vi "一致性结果判定.vi"() -> (14 "1":bool=TRUE, 15 "2":bool=TRUE, 16 "3":bool=TRUE, 17 "4":bool=TRUE, 18 "5":bool=TRUE, 19 "6":bool=TRUE)   [LabVIEW 2017]
panel:
  out "添加的数组 2":u32[](array[numeric])
  out "数组":bool[](array[boolean])
  in  "位置范围设定":T1={"位置1"={"上限"=726.0, "下限"=686.0}, "位置2"={"上限"=874.0, "下限"=834.0}, "位置3"={"上限"=997.0, "下限"=957.0}, "位置4"={"上限"=1139.0, "下限"=1099.0}, "位置5"={"上限"=1283.0, "下限"=1243.0}, "位置6"={"上限"=1429.0, "下限"=1389.0}, "位置7"={"上限"=1576.0, "下限"=1536.0}, "位置8"={"上限"=1728.0, "下限"=1688.0}, "位置9"={"上限"=1879.0, "下限"=1839.0}, "位置10"={"上限"=2036.0, "下限"=1996.0}}
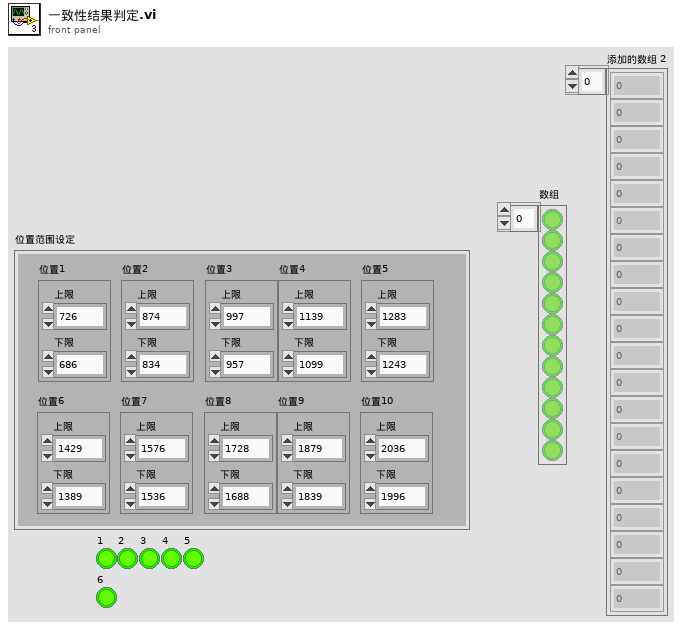
[diagram p1: front panel]
types:
  T1 = cluster{"位置1":cluster{"上限":dbl, "下限":dbl}, "位置2":cluster{"上限":dbl, "下限":dbl}, "位置3":cluster{"上限":dbl, "下限":dbl}, "位置4":cluster{"上限":dbl, "下限":dbl}, "位置5":cluster{"上限":dbl, "下限":dbl}, "位置6":cluster{"上限":dbl, "下限":dbl}, "位置7":cluster{"上限":dbl, "下限":dbl}, "位置8":cluster{"上限":dbl, "下限":dbl}, "位置9":cluster{"上限":dbl, "下限":dbl}, "位置10":cluster{"上限":dbl, "下限":dbl}}
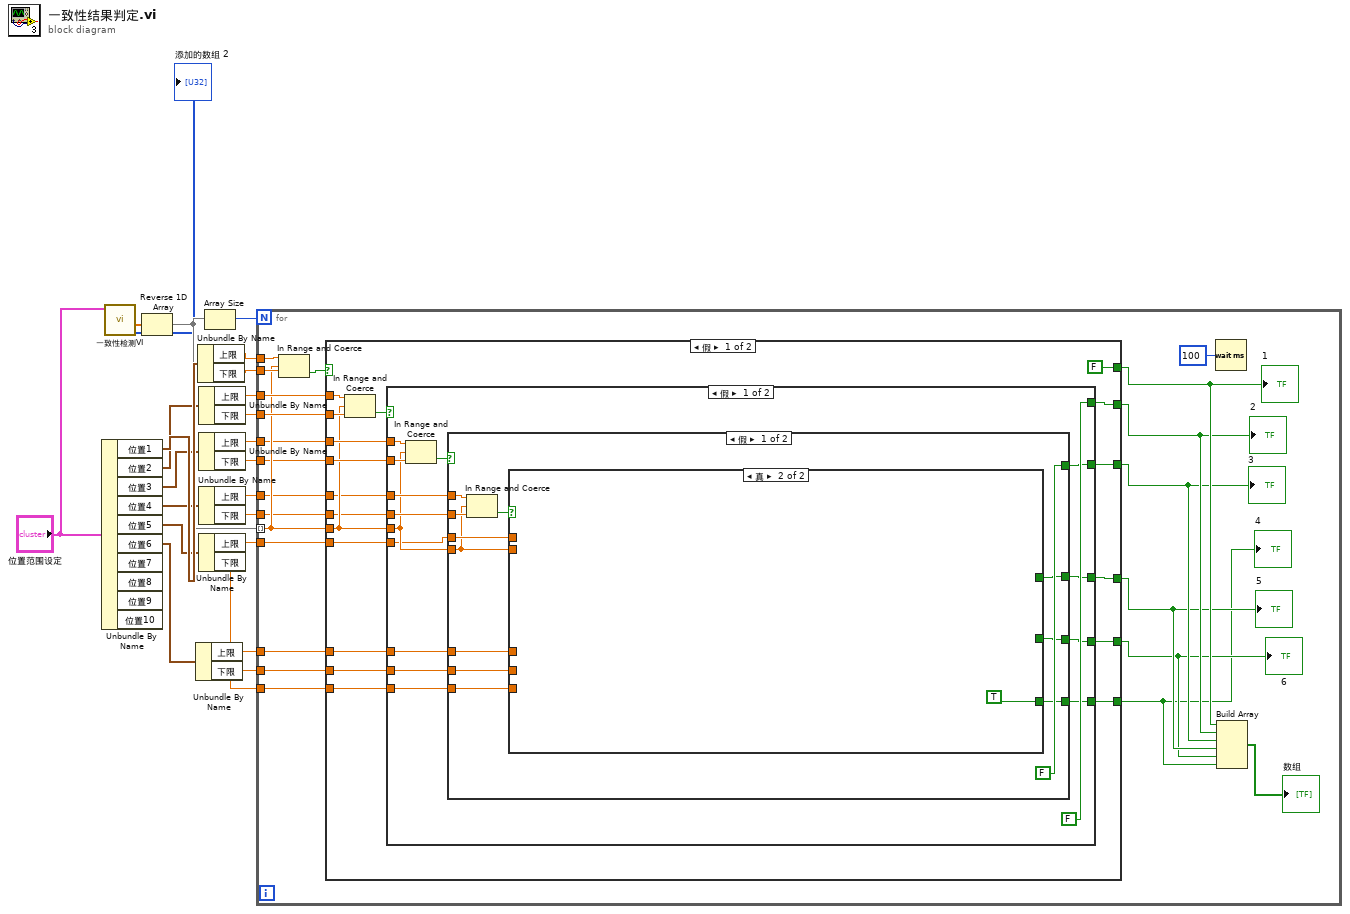
[diagram p0: block diagram]
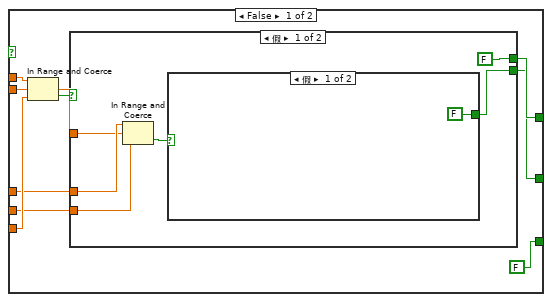
[diagram p2: hidden frame]
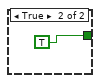
[diagram p3: hidden frame]
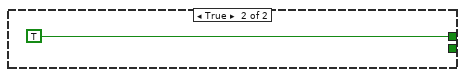
[diagram p4: hidden frame]
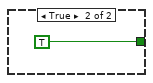
[diagram p5: hidden frame]
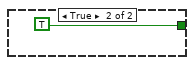
[diagram p6: hidden frame]
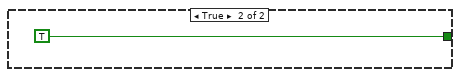
[diagram p7: hidden frame]
diagram:
  n1 = Unbundle By Name("位置范围设定") -> ("位置1"=w23:cluster{"上限":dbl, "下限":dbl}, "位置2"=w18:cluster{"上限":dbl, "下限":dbl}, "位置3"=w15:cluster{"上限":dbl, "下限":dbl}, "位置4"=w12:cluster{"上限":dbl, "下限":dbl}, "位置5"=w9:cluster{"上限":dbl, "下限":dbl}, "位置6"=w6:cluster{"上限":dbl, "下限":dbl})  [unwired: 4 out]
  n2 = call "一致性检测VI.vi"("位置范围设定"="位置范围设定") -> ("添加的数组 2"=→"添加的数组 2":u32[], "添加的数组"=w21:sgl[])  [unwired: 7 in, 2 out]
  n3 = Reverse 1D Array(array=w21) -> (reversed array=w2:sgl[])
  n4 = Unbundle By Name(w6) -> ("上限"=w5:dbl, "下限"=w4:dbl)
  n5 = Unbundle By Name(w23) -> ("上限"=w19:dbl, "下限"=w20:dbl)
  n6 = Unbundle By Name(w18) -> ("上限"=w16:dbl, "下限"=w17:dbl)
  n7 = Unbundle By Name(w15) -> ("上限"=w14:dbl, "下限"=w13:dbl)
  n8 = Unbundle By Name(w12) -> ("上限"=w11:dbl, "下限"=w10:dbl)
  n9 = Unbundle By Name(w9) -> ("上限"=w8:dbl, "下限"=w7:dbl)
  n10 = Array Size(array=w2) -> (size(s)=w22:i32)
  n11 = for {
    N: w22 -> [_]
    tunnel: w2 -> [w40] mode=indexing
    tunnel: w20 -> [w45]
    tunnel: w19 -> [w44]
    tunnel: w17 -> [w42]
    tunnel: w16 -> [w41]
    tunnel: w14 -> [w39]
    tunnel: w13 -> [w38]
    tunnel: w11 -> [w37]
    tunnel: w10 -> [w36]
    tunnel: w8 -> [w35]
    tunnel: w7 -> [w34]
    tunnel: w5 -> [w33]
    tunnel: w4 -> [w32]
    n12 = In Range and Coerce(upper limit=w44, x=w40, lower limit=w45) -> (In Range?=w43:bool)  [unwired: 1 out]
    n13 = case shown="假" w43 {
      tunnel: [FALSE ("1") TRUE ("1")] -> w30
      tunnel: w42 -> [w62 _]
      tunnel: w41 -> [w61 _]
      tunnel: w40 -> [w56 _]
      tunnel: [w59 _] -> w29
      tunnel: w39 -> [w58 _]
      tunnel: w38 -> [w57 _]
      tunnel: [w55 _] -> w28
      tunnel: w37 -> [w54 _]
      tunnel: w36 -> [w53 _]
      tunnel: [w52 _] -> w25
      tunnel: w35 -> [w51 _]
      tunnel: w34 -> [w50 _]
      tunnel: [w49 _] -> w27
      tunnel: w33 -> [w48 _]
      tunnel: w32 -> [w47 _]
      tunnel: [w46 _] -> w26
      frame False {
        n14 = In Range and Coerce(upper limit=w61, x=w56, lower limit=w62) -> (In Range?=w60:bool)  [unwired: 1 out]
        n15 = case shown="假" w60 {
          tunnel: [FALSE TRUE] -> w59
          tunnel: w58 -> [w76 _]
          tunnel: w57 -> [w75 _]
          tunnel: w56 -> [w71 _]
          tunnel: [w74 _] -> w55
          tunnel: w54 -> [w73 _]
          tunnel: w53 -> [w72 _]
          tunnel: [w70 _] -> w52
          tunnel: w51 -> [w69 _]
          tunnel: w50 -> [w68 _]
          tunnel: [w67 _] -> w49
          tunnel: w48 -> [w66 _]
          tunnel: w47 -> [w65 _]
          tunnel: [w64 _] -> w46
          frame False {
            n16 = In Range and Coerce(upper limit=w76, x=w71, lower limit=w75) -> (In Range?=w77:bool)  [unwired: 1 out]
            n17 = case shown="假" w77 {
              tunnel: [FALSE TRUE] -> w74
              tunnel: w73 -> [w88 _]
              tunnel: w72 -> [w87 _]
              tunnel: w71 -> [w82 _]
              tunnel: [w86 _] -> w70
              tunnel: w69 -> [w85 _]
              tunnel: w68 -> [w84 _]
              tunnel: [w83 _] -> w67
              tunnel: w66 -> [w81 _]
              tunnel: w65 -> [w80 _]
              tunnel: [w79 _] -> w64
              frame False {
                n18 = In Range and Coerce(upper limit=w88, x=w82, lower limit=w87) -> (In Range?=w89:bool)  [unwired: 1 out]
                n19 = case shown="真" w89 {
                  tunnel: [FALSE TRUE] -> w86
                  tunnel: w85 -> [w97 _]
                  tunnel: w84 -> [w96 _]
                  tunnel: [w95 _] -> w83
                  tunnel: w82 -> [w92 _]
                  tunnel: w81 -> [w94 _]
                  tunnel: w80 -> [w93 _]
                  tunnel: [w91 _] -> w79
                  frame False {
                    n20 = In Range and Coerce(upper limit=w97, x=w92, lower limit=w96) -> (In Range?=w98:bool)  [unwired: 1 out]
                    n21 = case shown="假" w98 {
                      tunnel: [FALSE TRUE] -> w95
                      tunnel: w94 -> [w103 _]
                      tunnel: w93 -> [w102 _]
                      tunnel: w92 -> [w101 _]
                      tunnel: [w100 _] -> w91
                      frame False {
                        n22 = In Range and Coerce(upper limit=w103, x=w101, lower limit=w102) -> (In Range?=w104:bool)  [unwired: 1 out]
                        n23 = case shown="假" w104 {
                          tunnel: [FALSE TRUE] -> w100
                          frame False {
                          }
                          frame True {
                          }
                        }
                      }
                      frame True {
                      }
                    }
                  }
                  frame True {
                  }
                }
              }
              frame True {
              }
            }
          }
          frame True {
          }
        }
      }
      frame True {
      }
    }
    "1" <- w30
    "2" <- w29
    "3" <- w28
    "4" <- w25
    "5" <- w27
    "6" <- w26
    n24 = Wait (ms)(milliseconds to wait=u32 100 ("等待时间（毫秒）")) -> ()  [unwired: 1 out]
    n25 = Build Array(w30, w29, w28, w27, w26, w25) -> (→"数组":bool[])
  }
